vi "mouse.vi"() -> ()   [LabVIEW 2020]
uses:
  <vilib>/Utility/inputDevices.llb/mouseAcquire.vi
  <vilib>/Utility/inputDevices.llb/closeMouse.vi
panel:
  in  "y":bool
  out "Vertical":i32
  out "Horizontal":i32
  out "button 2":bool
  out "button 1":bool
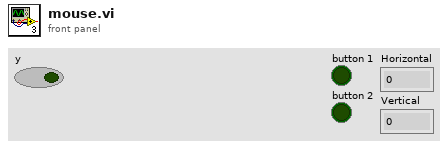
[diagram p1: front panel]
types:
  T1 = cluster{"Horizontal":i32, "Vertical":i32, "Scrolling":i32}
  T2 = cluster{"button 1":bool, "button 2":bool, "button 3":bool, "button 4":bool}
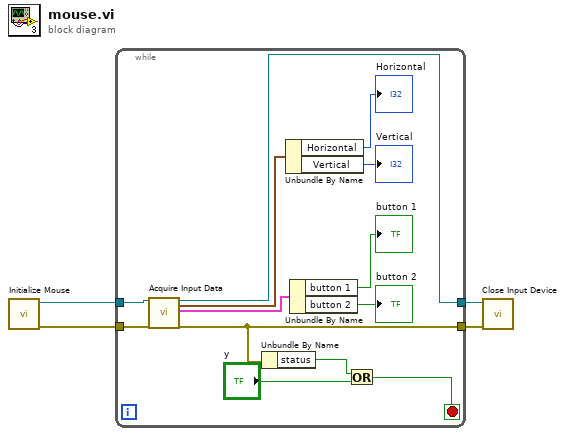
[diagram p0: block diagram]
diagram:
  n1 = call <vilib>:"Initialize Mouse.vi"() -> ("error out"=w2:errorcluster, "device ID"=w4:refnum<k1>)  [unwired: 10 in]
  n2 = while {
    tunnel: w4 -> [w17]
    tunnel: [w16] -> w3
    tunnel: w2 -> [w15]
    tunnel: [w8] -> w1
    stop <- w5 stop-if-true
    n3 = call-poly <vilib>:"Acquire Input Data.vi"("device ID"=w17, "error in (no error)"=w15) -> ("device ID"=w16:refnum<k1>, "axis info"=w14:T1, "button info"=w13:T2, "error out"=w8:errorcluster)  [unwired: 14 in]
    n4 = Unbundle By Name(w8) -> ("status"=w7:bool)
    n5 = Unbundle By Name(w14) -> ("Horizontal"=→"Horizontal":i32, "Vertical"=→"Vertical":i32)
    n6 = Unbundle By Name(w13) -> ("button 1"=→"button 1":bool, "button 2"=→"button 2":bool)
    n7 = Or(x=w7, y="y") -> (x .or. y?=w5:bool)
  }
  n8 = call-poly <vilib>:"Close Input Device.vi"("error in (no error)"=w1, "device ID"=w3) -> ()  [unwired: 8 in, 1 out]
